vi "UserDefinedPath.vi"() -> (3 "UserDefinedPath":T1={"TREE PNG"=path "", "User Guide"=path "", "DefaultSave"=path "", "BuildPath"=path "", "Image"=path "", "Modules"=path "", "Configuration"=path "", "License"=path "I:/0. iAmleoCHO/0.09 Projects_ZCJX/2017/3. 6Y11S_ZMS_液流台&热气台数据采集/ZcDAQ/E/LabviewPrj/曹队/ZcDAQprj/Modules/DAQ-Device/Hardware Drivers/QX/HBM LabVIEW Driver/DLLs/HBM LabVIEW Driver.license", "SplitFiles"=path "I:/0. iAmleoCHO/0.09 Projects_ZCJX/2017/3. 6Y11S_ZMS_液流台&热气台数据采集/ZcDAQ/E/LabviewPrj/曹队/ZcDAQprj/Modules/DAQ-Device/Hardware Drivers/QX/HBM LabVIEW Driver/DLLs/HBM LabVIEW Driver.license", "System.ini"=path ""})   [LabVIEW 2016]
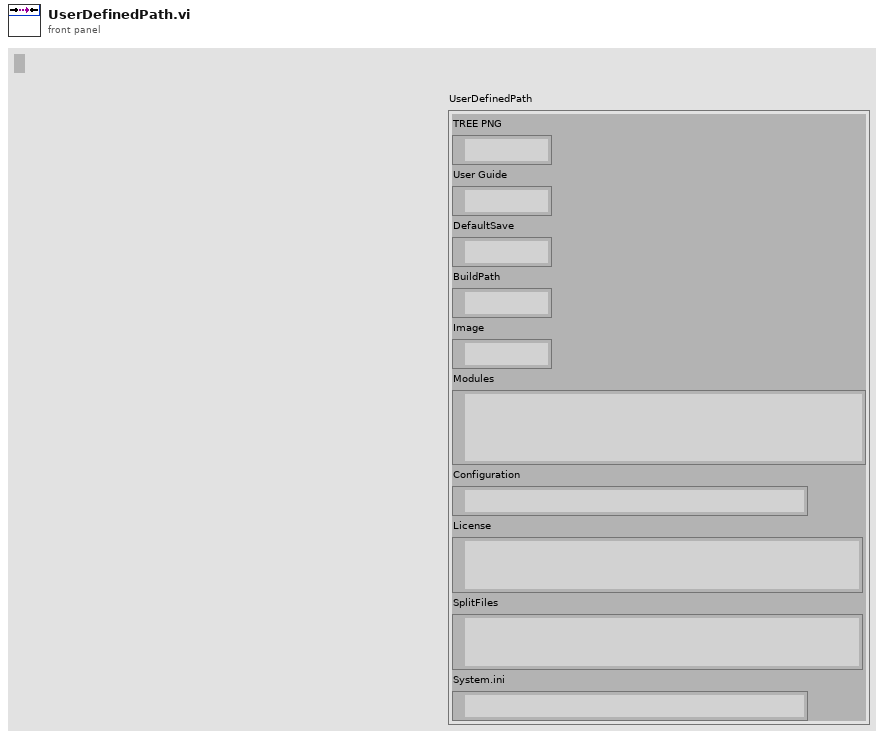
[diagram p1: front panel]
types:
  T1 = cluster{"TREE PNG":path, "User Guide":path, "DefaultSave":path, "BuildPath":path, "Image":path, "Modules":path, "Configuration":path, "License":path, "SplitFiles":path, "System.ini":path}
  T2 = enum32{"invalid app kind", "Development System", "Run Time System", "Student Edition", "Embedded LabVIEW", "Evaluation", "Custom"}
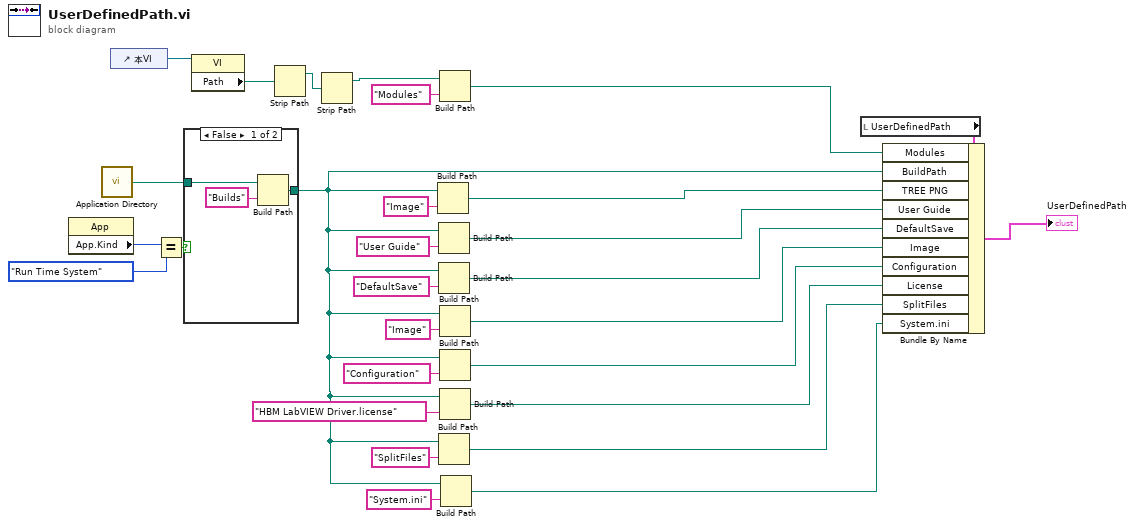
[diagram p0: block diagram]
diagram:
  n1 = property class="App"() -> ("App.Kind"=w26:T2)  [unwired: 2 in, 2 out]
  n2 = call <vilib>:"Application Directory.vi"() -> ("Application Directory"=w29:path)
  n3 = control-ref of="本VI"() -> (w16:refnum<vi>)
  n4 = Equal?(x=w26, y=T2."Run Time System") -> (x = y?=w24:bool)
  n5 = case shown="False" w24 {
    tunnel: w29 -> [w32 w33]
    tunnel: [w30 w33] -> w2
    frame False {
      n6 = Build Path(base path=w32, name or relative path="Builds" ("名称或相对路径")) -> (appended path=w30:path)
    }
    frame True {
    }
  }
  n7 = property class="VI"(reference=w16) -> ("Path"=w15:path)  [unwired: 1 in, 2 out]
  n8 = Strip Path(path=w15) -> (stripped path=w14:path)  [unwired: 1 out]
  n9 = Strip Path(path=w14) -> (stripped path=w8:path)  [unwired: 1 out]
  n10 = Build Path(base path=w2, name or relative path="Image" ("名称或相对路径")) -> (appended path=w22:path)
  n11 = Build Path(base path=w2, name or relative path="User Guide" ("名称或相对路径")) -> (appended path=w20:path)
  n12 = Build Path(base path=w2, name or relative path="DefaultSave" ("名称或相对路径")) -> (appended path=w18:path)
  n13 = Build Path(base path=w2, name or relative path="SplitFiles" ("名称或相对路径")) -> (appended path=w5:path)
  n14 = Build Path(base path=w8, name or relative path="Modules" ("名称或相对路径")) -> (appended path=w6:path)
  n15 = Build Path(base path=w2, name or relative path="Image" ("名称或相对路径")) -> (appended path=w11:path)
  n16 = Build Path(base path=w2, name or relative path="Configuration" ("名称或相对路径")) -> (appended path=w10:path)
  n17 = Build Path(base path=w2, name or relative path="HBM LabVIEW Driver.license" ("名称或相对路径")) -> (appended path=w7:path)
  n18 = Build Path(base path=w2, name or relative path="System.ini" ("名称或相对路径")) -> (appended path=w1:path)
  n19 = local read "UserDefinedPath"() -> (w28:T1)
  n20 = Bundle By Name(cluster=w28, "Modules"=w6, "BuildPath"=w2, "TREE PNG"=w22, "User Guide"=w20, "DefaultSave"=w18, "Image"=w11, "Configuration"=w10, "License"=w7, "SplitFiles"=w5, "System.ini"=w1) -> (→"UserDefinedPath":T1)
